vi "Start Counting.vi"(8 "error in (no error)":errorcluster, 10 "Duration":dbl, 11 "Timer in":refnum<class "Timer.lvclass">) -> (0 "error out":errorcluster, 3 "Timer out":refnum<class "Timer.lvclass">)   [LabVIEW 2024, in "Timer.lvlib" / "Timer.lvclass"]
uses:
  Timer.lvclass
  Timer.lvclass/Timer.ctl
  <vilib>/ActorFramework/Actor/Actor.lvclass
  Chef Actor Logic/Chef Actor Logic Messages/Update Elapsed Time Msg/Update Elapsed Time Msg.lvclass
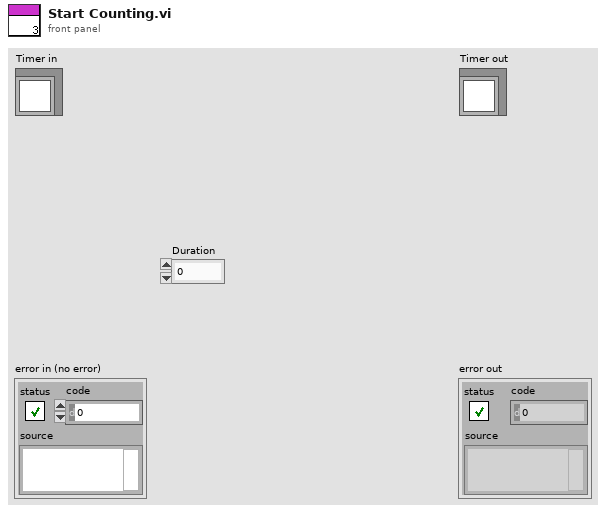
[diagram p1: front panel]
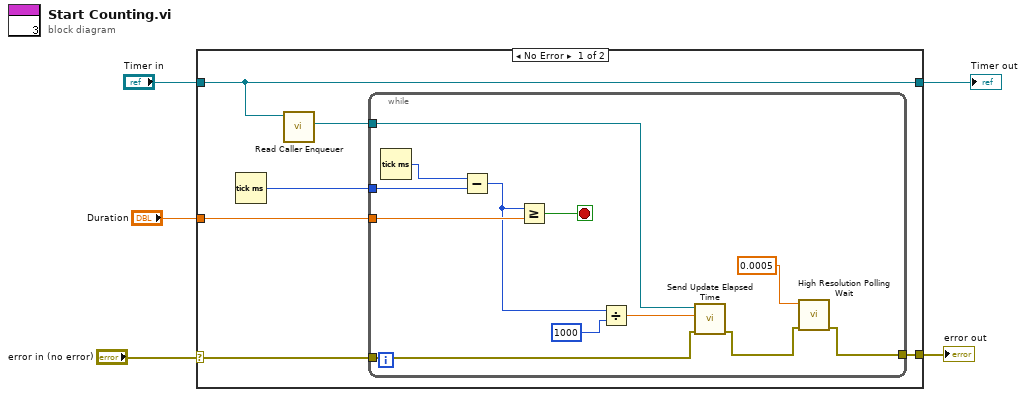
[diagram p0: block diagram]
diagram:
  n1 = case shown="No Error" "error in (no error)" {
    selector: "error in (no error)" -> [w8 w25]
    tunnel: [w7 w25] -> w4
    tunnel: [w10 w24] -> w2
    tunnel: "Timer in" -> [w10 w24]
    tunnel: "Duration" -> [w6 _]
    frame No Error {
      n2 = Tick Count (ms)() -> (millisecond timer value=w11:u32)
      n3 = call <vilib>:"Read Caller Enqueuer.vi"("Actor"=w10) -> ("Caller Enqueuer"=w9:refnum<class "Message Enqueuer.lvclass">)  [unwired: 10 in]
      n4 = while {
        tunnel: w11 -> [w22]
        tunnel: w6 -> [w21]
        tunnel: w9 -> [w15]
        tunnel: w8 -> [w14]
        tunnel: [w17] -> w7
        stop <- w20 stop-if-true
        n5 = Tick Count (ms)() -> (millisecond timer value=w23:u32)
        n6 = Subtract(x=w23, y=w22) -> (x-y=w19:u32)
        n7 = Greater Or Equal?(x=w19, y=w21) -> (x >= y?=w20:bool)
        n8 = Divide(x=w19, y=u32 1000) -> (x/y=w13:dbl)
        n9 = call "Send Update Elapsed Time.vi"("error in (no error)"=w14, "Elapsed Time"=w13, "Message Enqueuer"=w15) -> ("error out"=w12:errorcluster)  [unwired: 7 in, 1 out]
        n10 = call <vilib>:"High Resolution Polling Wait.vi"("error in (no error)"=w12, "seconds to wait"=0.0005) -> ("error out"=w17:errorcluster)  [unwired: 9 in]
      }
    }
    frame Error {
    }
  }
  "error out" <- w4
  "Timer out" <- w2
